vi "zero_set.vi"(11 "Array in":dbl[](array[numeric])) -> (3 "Array out":dbl[](array[numeric]))   [LabVIEW 2020]
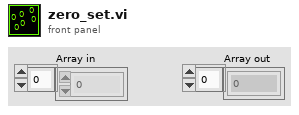
[diagram p1: front panel]
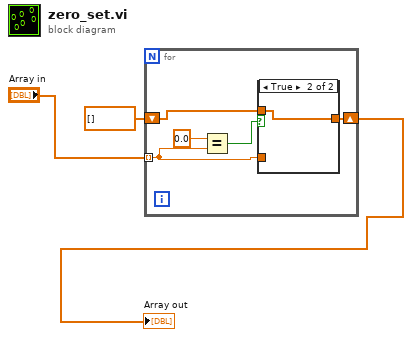
[diagram p0: block diagram]
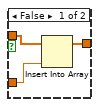
[diagram p2: hidden frame]
diagram:
  n1 = for {
    tunnel: "Array in" -> [w7] mode=indexing
    shift-right: [w5] -> w3
    shift-left: dbl[] [] -> [w4]
    n2 = Equal?(x=0.0, y=w7) -> (x = y?=w8:bool)
    n3 = case shown="True" w8 {
      tunnel: w7 -> [w11 _]
      tunnel: [w10 w12] -> w5
      tunnel: w4 -> [w9 w12]
      frame False {
        n4 = Insert Into Array(array=w9, new element=w11) -> (w10:dbl[])  [unwired: 1 in]
      }
      frame True {
      }
    }
  }
  "Array out" <- w3
